vi "Zadanie 4.vi"() -> ()   [LabVIEW 2020]
panel:
  out "number 2":u32
  in  "Boolean":bool
  out "number":u32
  out "Array 2":bool[](array[boolean])
  in  "Array":bool[](array[boolean])
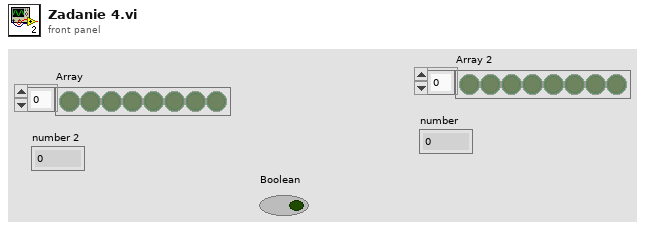
[diagram p1: front panel]
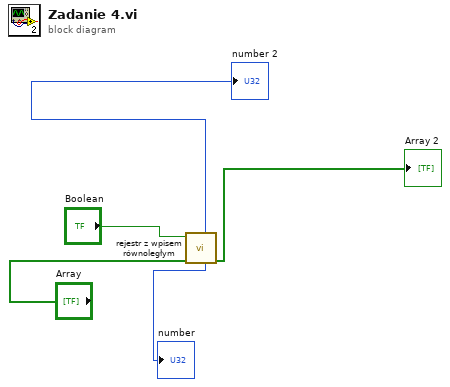
[diagram p0: block diagram]
diagram:
  n1 = call "rejestr z wpisem równoległym.vi"("Wejście danych"="Array", "Switch"="Boolean") -> ("Wyjście danych"=→"Array 2":bool[], "zliczenia wyjścia"=→"number":u32, "zalicenia wejścia"=→"number 2":u32)  [unwired: 7 in]
